vi "fdyukfggchk.vi"() -> ()   [LabVIEW 2016]
uses:
  Get Motor Temperature Config.vi
  <vilib>/CANopenLib/CANOPEN.llb/CANopen SDO Create.vi
  <vilib>/CANopenLib/CANOPEN.llb/CANopen SDO Write [I32].vi
  <vilib>/CANopenLib/CANOPEN.llb/CANopen SDO Read [Block].vi
panel:
  out "Motor Temperature Config":T1
  in  "Node ID":u8 min=1 max=127 step=1
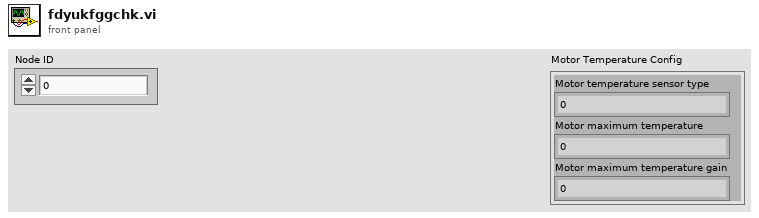
[diagram p1: front panel]
types:
  T1 = cluster{"Motor temperature sensor type":u8, "Motor maximum temperature":u8, "Motor maximum temperature gain":i16}
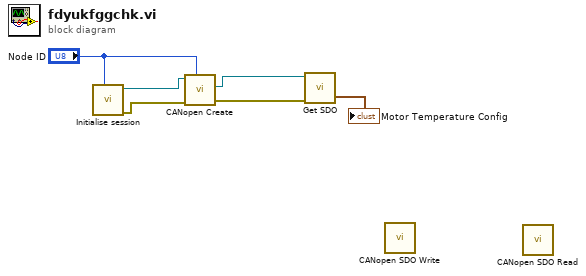
[diagram p0: block diagram]
diagram:
  n1 = call "Initialise session.vi"("Node ID"="Node ID") -> ("error out"=w3:errorcluster, "interface object out"=w4:refnum<k20>)  [unwired: 8 in, 1 out]
  n2 = call-poly <vilib>:"CANopen Create.vi"("node-ID"="Node ID", "error in (no error)"=w3, "interface object in"=w4) -> ("error out"=w5:errorcluster, "SDO object out"=w6:refnum<k20>)  [unwired: 6 in, 1 out]
  n3 = call-poly "Get SDO.vi"("error in (no error)"=w5, "SDO object in"=w6) -> ("Motor Temperature Config"=→"Motor Temperature Config":T1)  [unwired: 6 in, 3 out]
  n4 = call-poly <vilib>:"CANopen SDO Write.vi"() -> ()  [unwired: 9 in, 3 out]
  n5 = call-poly <vilib>:"CANopen SDO Read.vi"() -> ()  [unwired: 8 in, 4 out]
